vi "Prompt for Step--UI Interlocks.vi"(8 "error in (no error)":errorcluster, 10 "Control Ref Map":map{string, refnum<vi>}(c390), 11 "String Assertion in":refnum<class "String Assertion.lvclass">) -> (0 "error out":errorcluster, 2 "Error List":string[](array[string]), 3 "String Assertion out":refnum<class "String Assertion.lvclass">)   [LabVIEW 2020, in "MacroAssert.lvlib" / "String Assertion.lvclass"]
doc: "Enables or disables buttons within the \"Prompt for Step\" VI according to the current state of the system."
uses:
  String Assertion.lvclass
  C:/Users/User/Documents/LabVIEW Data/Projects/MacroAssert/source/Classes/Assertion Step/Assertion Step.lvclass
  String Assertion Type.ctl
  Support/Get Control Reference by Label (1D STR).vi
  MacroAssert.lvlib
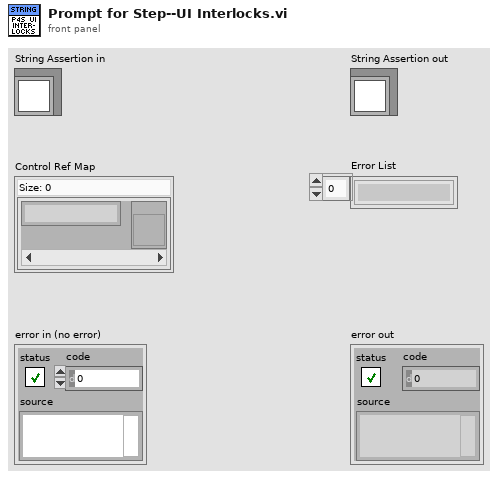
[diagram p1: front panel]
types:
  T1 = typedef "MacroAssert.lvlib/String Assertion.lvclass/String Assertion Type.ctl" = enum16{"String Ctl Value", "Ctl Caption Property", "Ctl Tip Strip Property", "Frontmost VI Name", "Frontmost Window Name"}
  T2 = enum8{"Enabled", "Disabled", "Disabled and Grayed Out"}
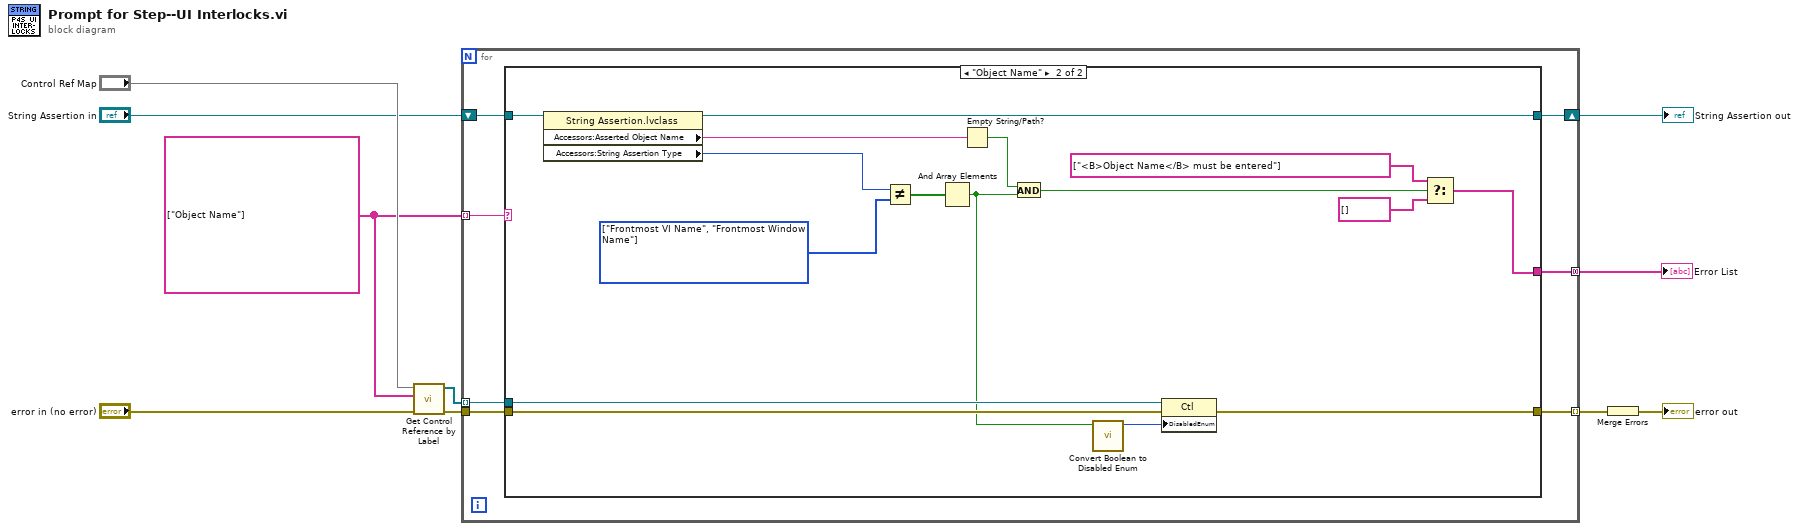
[diagram p0: block diagram]
diagram:
  w5 = string[] ["Object Name"]
  n1 = call-poly "Get Control Reference by Label.vi"("error in (no error)"="error in (no error)", "Control Names"=w5, "Control Ref Map"="Control Ref Map") -> ("error out"=w7:errorcluster, "Control Refs"=w6:refnum<vi>[])  [unwired: 6 in, 1 out]
  n2 = for {
    shift-right: [w14] -> w2
    shift-left: "String Assertion in" -> [w17]
    tunnel: w5 -> [w16] mode=indexing
    tunnel: [w15] -> w3 mode=indexing
    tunnel: w7 -> [w13]
    tunnel: w6 -> [w12] mode=indexing
    tunnel: [w11] -> w1 mode=concatenating
    n3 = case shown="\"Object Name\"" w16 {
      tunnel: w17 -> [w18 w35]
      tunnel: w13 -> [w19 w33]
      tunnel: [w19 w32] -> w15
      tunnel: [w18 w34] -> w14
      tunnel: w12 -> [_ w31]
      tunnel: [_ w26] -> w11
      frame Default {
      }
      frame "Object Name" {
        w20 = T1[] [enum."Frontmost VI Name", enum."Frontmost Window Name"] items=["String Ctl Value", "Ctl Caption Property", "Ctl Tip Strip Property", "Frontmost VI Name", "Frontmost Window Name"]
        n4 = property class="String Assertion.lvclass"(reference=w35) -> (reference out=w34:refnum<class "String Assertion.lvclass">, "Accessors:Asserted Object Name"=w23:string, "Accessors:String Assertion Type"=w24:T1)  [unwired: 1 in, 1 out]
        n5 = Not Equal?(x=w24, y=w20) -> (x != y?=w30:bool[])
        n6 = And Array Elements(Boolean array=w30) -> (logical AND=w25:bool)
        n7 = Empty String/Path?(string/path=w23) -> (empty?=w22:bool)
        n8 = And(x=w22, y=w25) -> (x .and. y?=w21:bool)
        n9 = call "Convert Boolean to Disabled Enum.vi"("Enabled?"=w25) -> ("Disabled Enum"=w29:T2)  [unwired: 10 in]
        n10 = property class="Ctl"(reference=w31, error in=w33, "DisabledEnum"=w29) -> (error out=w32:errorcluster)  [unwired: 1 out]
        n11 = Select(t=string[] ["<B>Object Name</B> must be entered"], s=w21, f=string[] []) -> (s? t:f=w26:string[])
      }
    }
  }
  "String Assertion out" <- w2
  "Error List" <- w1
  n12 = Merge Errors(w3) -> (→"error out":errorcluster)
